vi "Teleop.vi"(10 "Match Info":T2={"Autonomous Elapsed Seconds"=0.0, "TeleOp Elapsed Seconds"=0.0, "Disabled Elapsed Seconds"=0.0, "Visited Autonomous"=FALSE, "Visited TeleOp"=FALSE, "Visited Disabled"=FALSE, "Autonomous Settings"={"Autonomous Style"=enum."Independent", "VI Refnum"=refnum}}, 11 "Call Context":T3) -> ()   [LabVIEW 2017]
doc: "This VI is called for each TeleOp packet received from the DS where the robot is not disabled. It is often used to read from the joysticks and update I/O or to update setpoints for timed control loops. It should complete and return within 20 milliseconds or it may miss DS packets."
uses:
  <vilib>/Rock Robotics/WPI/DriverStation/WPI_DriverStationDerivedRobotMode.ctl
  <vilib>/Rock Robotics/WPI/DriverStation/WPI_DriverStationMatch Info.ctl
  <vilib>/Rock Robotics/WPI/Solenoid/WPI_SolenoidValue.ctl
  <vilib>/Rock Robotics/WPI/Utilities/WPI_GetSetVariantRefNum.vi
  <vilib>/Rock Robotics/WPI/RobotDrive/WPI_RobotDriveMecanumDrive_Cartesian.vi
  <vilib>/Rock Robotics/Network Tables/NT Write Numeric Array.vi
  <vilib>/Rock Robotics/WPI/Solenoid/WPI_SolenoidSetEnum.vi
  Robot Global Data.vi
  <vilib>/Rock Robotics/Network Tables/NT Write Number.vi
panel:
  out "Stopped":bool
  out "Rate":dbl
  out "Direction":bool
  out "Distance":dbl
  out "Accelerations":T1
  out "Switch Pressed":bool
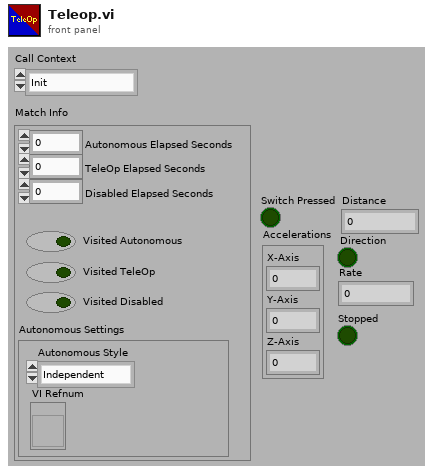
[diagram p1: front panel]
types:
  T1 = cluster{"X-Axis":dbl, "Y-Axis":dbl, "Z-Axis":dbl}
  T2 = typedef "WPI_DriverStationMatch Info.ctl" = cluster{"Autonomous Elapsed Seconds":dbl, "TeleOp Elapsed Seconds":dbl, "Disabled Elapsed Seconds":dbl, "Visited Autonomous":bool, "Visited TeleOp":bool, "Visited Disabled":bool, "Autonomous Settings":cluster{"Autonomous Style":enum16{"Iterative", "Independent"}, "VI Refnum":refnum<vi>}}
  T3 = typedef "WPI_DriverStationDerivedRobotMode.ctl" = enum16{"Init", "Execute", "Stop"}
  T4 = typedef "WPI_SolenoidValue.ctl" = enum16{"Off", "On", "Forward", "Reverse"}
  T5 = typedef "WPI_JoystickDevRef.ctl" = cluster{"Device":T6}
  T6 = typedef "WPI_JoystickDeviceEnum.ctl" = enum16{"USB 0", "USB 1", "USB 2", "USB 3", "USB 4", "USB 5"}
  T7 = typedef "WPI_MotorControlDeviceRef.ctl" = cluster{"DeviceStatus":errorcluster, "Type":T8, "PWM":cluster{"PWM Channel":T9, "DeadBand":T10}, "CAN":cluster{"Device Number":u8, "SetOutput VI Ref":variant, "GetOutput VI Ref":variant, "Enable VI Ref":variant, "Disable VI Ref":variant, "Data":variant}, "Invert":bool, "DIO PWM":cluster{"PWM \"Enable\" Channel":T9, "DIOChannel":T11, "PWM Rate":dbl}}
  T8 = typedef "WPI_MotorControlType.ctl" = enum16{"PWM", "CAN", "DIO PWM"}
  T9 = typedef "FPGA_DIOPWMChannel.ctl" = enum8{"PWM 0", "PWM 1", "PWM 2", "PWM 3", "PWM 4", "PWM 5", "PWM 6", "PWM 7", "PWM 8", "PWM 9", "PWM MXP 0", "PWM MXP 1", "PWM MXP 2", "PWM MXP 3", "PWM MXP 4", "PWM MXP 5", "PWM MXP 6", "PWM MXP 7", "PWM MXP 8", "PWM MXP 9", "Invalid"}
  T10 = typedef "WPI_PWMDeadband.ctl" = cluster{"Name":string, "maxPositivePwm":i32, "minPositivePwm":i32, "centerPwm":i32, "maxNegativePwm":i32, "minNegativePwm":i32, "angularRange":u16}
  T11 = typedef "FPGA_DIOChannel.ctl" = enum8{"DIO 0", "DIO 1", "DIO 2", "DIO 3", "DIO 4", "DIO 5", "DIO 6", "DIO 7", "DIO 8", "DIO 9", "DIO MXP 0", "DIO MXP 1", "DIO MXP 2", "DIO MXP 3", "DIO MXP 4", "DIO MXP 5", "DIO MXP 6", "DIO MXP 7", "DIO MXP 8", "DIO MXP 9", "DIO MXP 10", "DIO MXP 11", "DIO MXP 12", "DIO MXP 13", "DIO MXP 14", "DIO MXP 15", "SPI Port CS1", "SPI Port CS2", "SPI Port CS3", "SPI Port MISO", "SPI Port MOSI", "Invalid"}
  T12 = typedef "WPI_SolenoidDevRef.ctl" = cluster{"DevStatus":errorcluster, "Pneumatics Control Module":u8, "Forward Solenoid Channel":T13, "Reverse Solenoid Channel":T13}
  T13 = typedef "WPI_SolenoidChannel.ctl" = enum8{"Solenoid 0", "Solenoid 1", "Solenoid 2", "Solenoid 3", "Solenoid 4", "Solenoid 5", "Solenoid 6", "Solenoid 7", "Invalid"}
  T14 = typedef "WPI_RobotDriveDevRef.ctl" = cluster{"DevStatus":errorcluster, "Motors[]":T7[], "Square Inputs":bool, "Max Output":dbl}
  T15 = typedef "WPI_SwitchDevRef.ctl" = cluster{"DevStatus":errorcluster, "DIO Channel":T11, "CntIndex":T16, "Normally Closed":bool}
  T16 = typedef "FPGA_CounterCtrSystemIndex.ctl" = enum8{"Ctr 0", "Ctr 1", "Ctr 2", "Ctr 3", "Ctr 4", "Ctr 5", "Ctr 6", "Ctr 7", "Invalid"}
  T17 = typedef "WPI_AccelerometerDevRef.ctl" = cluster{"DevStatus":errorcluster, "Scaling":T18, "Analog Channels":T19, "I2C Bus":T21, "SPI Bus":T22, "Accel Range":T23, "ADXL Axes":T24, "Handle":i32, "Device Address":u8, "Accel Type":enum16{"Analog", "ADXL345 I2C", "ADXL345 SPI", "Internal", "ADXL362 SPI"}}
  T18 = typedef "WPI_AccelerometerScaling.ctl" = cluster{"Gain (VoltsPerG)":dbl, "Center Voltage":dbl}
  T19 = typedef "WPI_AccelerometerAnalogChannels.ctl" = cluster{"X-Axis":T20, "Y-Axis":T20, "Z-Axis":T20}
  T20 = typedef "FPGA_AIChannel.ctl" = enum8{"AI 0", "AI 1", "AI 2", "AI 3", "AI MXP 0", "AI MXP 1", "AI MXP 2", "AI MXP 3", "Invalid"}
  T21 = typedef "i2c_bus.ctl" = enum16{"I2C On-Board", "I2C MXP", "Invalid"}
  T22 = typedef "spi_bus.ctl" = enum16{"SPI On-Board, CS0", "SPI On-Board, CS1", "SPI On-Board, CS2", "SPI On-Board, CS3", "SPI MXP", "Invalid"}
  T23 = typedef "ADXL345 Range.ctl" = u8
  T24 = typedef "WPI_AccelerometerADXL345 Axes.ctl" = cluster{"X-Axis":bool, "Y-Axis":bool, "Z-Axis":bool}
  T25 = typedef "WPI_EncoderDevRef.ctl" = cluster{"DevStatus":errorcluster, "EncoderIndex":T26, "CounterIndex":T16, "DistancePerCount":dbl, "Decoding Type":T27}
  T26 = typedef "FPGA_EncoderIdx.ctl" = enum8{"Enc 0", "Enc 1", "Enc 2", "Enc 3", "Enc 4", "Enc 5", "Enc 6", "Enc 7", "Invalid"}
  T27 = typedef "WPI_EncoderType.ctl" = enum16{"1x", "2x", "4x"}
  T28 = typedef "WPI_GyroDevRef.ctl" = cluster{"DevStatus":errorcluster, "Analog Channel":T20, "Gain (VoltsPerDegree/Second)":dbl, "Gyro Type":enum16{"Analog", "XRS450"}, "Handle":i32, "SPI Bus":T22, "Device Found":bool, "Sample Rate":dbl, "Calibrate On Open":bool, "Offset":dbl}
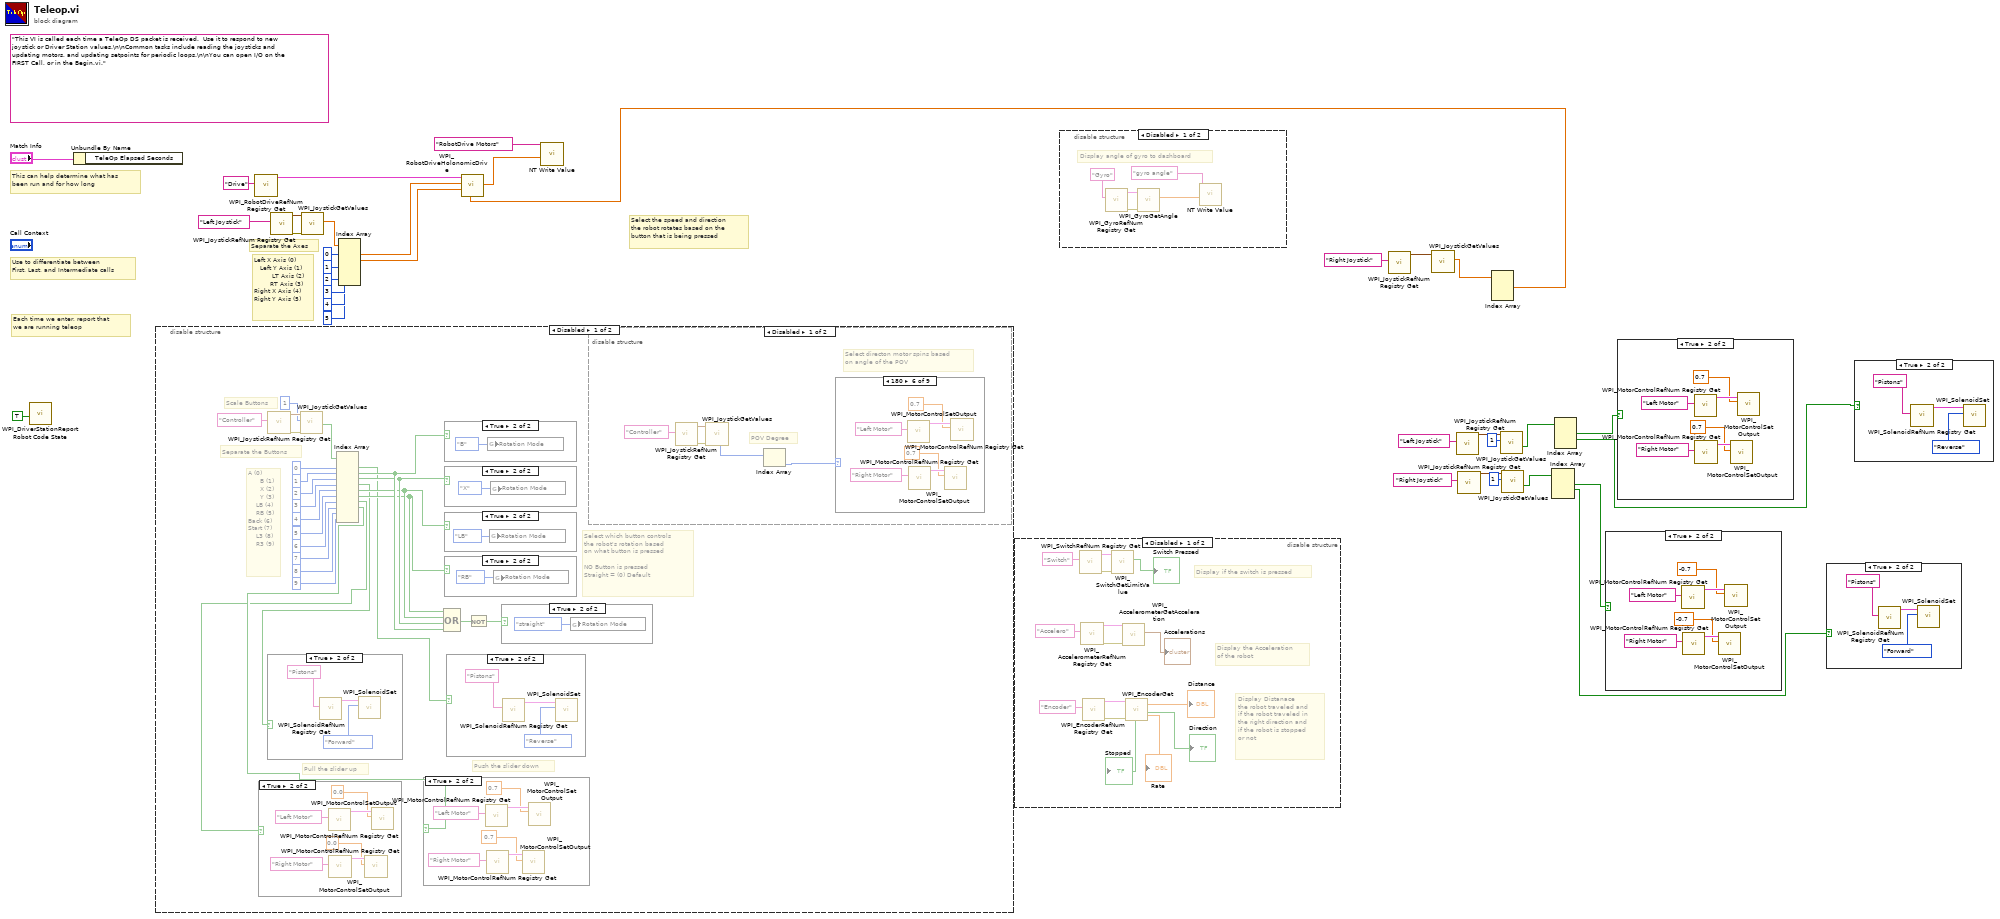
[diagram p0: block diagram]
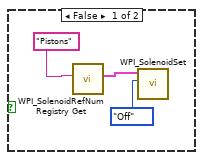
[diagram p2: hidden frame]
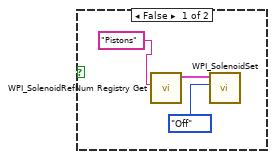
[diagram p3: hidden frame]
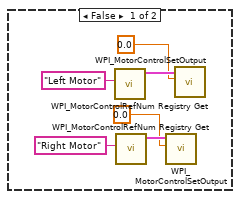
[diagram p4: hidden frame]
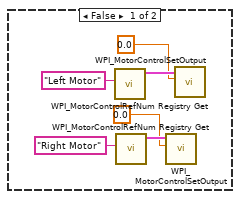
[diagram p5: hidden frame]
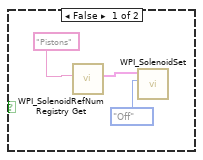
[diagram p8: hidden frame]
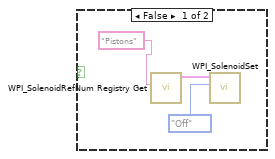
[diagram p9: hidden frame]
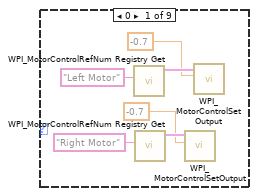
[diagram p15: hidden frame]
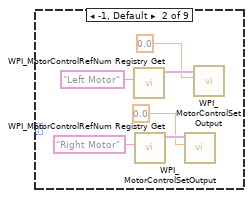
[diagram p16: hidden frame]
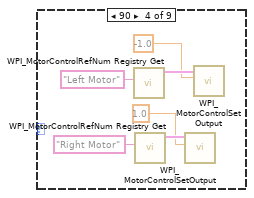
[diagram p18: hidden frame]
diagram:
  (unwired) "This VI is called each time a TeleOp DS packet is received.  Use it to respond to new joystick or Driver Station values.\n\nCommon tasks include reading the joysticks and updating motors, and updating setpoints for periodic loops.\n\nYou can open I/O on the FIRST Call, or in the Begin.vi."
  # "Select the speed and direction\nthe robot rotates based on the \nbutton that is being pressed"
  # "Left X Axis (0)\n   Left Y Axis (1)\n         LT Axis (2)\n        RT Axis (3)\nRight X Axis (4)\nRight Y Axis (5)"
  # "Separate the Axes"
  # "Each time we enter, report that\nwe are running teleop"
  # "Use to differentiate between\nFirst, Last, and Intermediate calls"
  # "This can help determine what has\nbeen run and for how long"
  n1 = call <vilib>:"WPI_DriverStationReport Robot Code State.vi"("TeleOp"=TRUE ("Autonomous")) -> ()  [unwired: 10 in, 1 out]
  n2 = Unbundle By Name("Match Info") -> ()  [unwired: 1 out]
  n3 = disable-structure shown="Disabled" {
    frame Disabled {
      # "Select which button controls\nthe robot's rotation based\non what button is pressed\n\nNO Button is pressed\nStraight = (0) Default"
      # "Pull the slider up"
      # "Push the slider down"
      # "A (0)\n      B (1)\n      X (2)\n      Y (3)\n    LB (4)\n    RB (5)\nBack (6)\nStart (7)\n    L3 (8)\n    R3 (9)"
      # "Separate the Buttons"
      # "Scale Buttons"
      n4 = call <vilib>:"WPI_JoystickRefNum Registry Get.vi"("refnum name"="Controller") -> ("error out"=w59:errorcluster, "JoystickDevRef"=w58:T5)  [unwired: 9 in]
      n5 = call <vilib>:"WPI_JoystickGetValues.vi"("error in (no error)"=w59, "Scaler"=i8 1, "JoystickDevRef"=w58) -> ("Buttons"=w37:bool[])  [unwired: 4 in, 4 out]
      n6 = Index Array(array=w37, index #1=0 ("index"), index #2=1 ("index"), index #3=2 ("index"), index #4=3 ("index"), index #5=4 ("index"), index #6=5 ("index"), index #7=6 ("index"), index #8=7 ("index"), index #9=8 ("index"), index #10=9 ("index")) -> (element #1=w39:bool, element #2=w43:bool, element #3=w42:bool, element #4=w38:bool, element #5=w41:bool, element #6=w40:bool, element #7=w35:bool, element #8=w36:bool)  [unwired: 2 out]
      n7 = case shown="True" w35 {
        frame False {
        }
        frame True {
          n8 = call <vilib>:"WPI_MotorControlRefNum Registry Get.vi"("refnum name"="Left Motor") -> ("MotorControlDevRef"=w70:T7)  [unwired: 9 in, 1 out]
          n9 = call <vilib>:"WPI_MotorControlRefNum Registry Get.vi"("refnum name"="Right Motor") -> ("MotorControlDevRef"=w71:T7)  [unwired: 9 in, 1 out]
          n10 = call <vilib>:"WPI_MotorControlSetOutput.vi"("Output"=0.0, "MotorControlDevRef"=w71) -> ()  [unwired: 7 in, 3 out]
          n11 = call <vilib>:"WPI_MotorControlSetOutput.vi"("Output"=0.0, "MotorControlDevRef"=w70) -> ()  [unwired: 7 in, 3 out]
        }
      }
      n12 = case shown="True" w38 {
        frame False {
          n13 = call <vilib>:"WPI_SolenoidRefNum Registry Get.vi"("refnum name"="Pistons") -> ("SolenoidDevRef"=w74:T12)  [unwired: 9 in, 1 out]
          n14 = call-poly <vilib>:"WPI_SolenoidSet.vi"("Value"=WPI_SolenoidValue."Off", "SolenoidDevRef"=w74) -> ()  [unwired: 8 in, 2 out]
        }
        frame True {
          n15 = call <vilib>:"WPI_SolenoidRefNum Registry Get.vi"("refnum name"="Pistons") -> ("SolenoidDevRef"=w76:T12)  [unwired: 9 in, 1 out]
          n16 = call-poly <vilib>:"WPI_SolenoidSet.vi"("Value"=WPI_SolenoidValue."Forward", "SolenoidDevRef"=w76) -> ()  [unwired: 8 in, 2 out]
        }
      }
      n17 = case shown="True" w36 {
        frame False {
        }
        frame True {
          n18 = call <vilib>:"WPI_MotorControlRefNum Registry Get.vi"("refnum name"="Left Motor") -> ("MotorControlDevRef"=w64:T7)  [unwired: 9 in, 1 out]
          n19 = call <vilib>:"WPI_MotorControlRefNum Registry Get.vi"("refnum name"="Right Motor") -> ("MotorControlDevRef"=w62:T7)  [unwired: 9 in, 1 out]
          n20 = call <vilib>:"WPI_MotorControlSetOutput.vi"("Output"=0.7, "MotorControlDevRef"=w62) -> ()  [unwired: 7 in, 3 out]
          n21 = call <vilib>:"WPI_MotorControlSetOutput.vi"("Output"=0.7, "MotorControlDevRef"=w64) -> ()  [unwired: 7 in, 3 out]
        }
      }
      n22 = Compound Arithmetic op=OR(w40, w41, w42, w43) -> (w55:bool)
      n23 = case shown="True" w43 {
        frame False {
        }
        frame True {
          n24 = global write "Robot Global Data.vi" "Rotation Mode"(enum16{"straight", "X", "LB", "B", "RB"}."B" ("Rotation Mode")) -> ()
        }
      }
      n25 = case shown="True" w42 {
        frame False {
        }
        frame True {
          n26 = global write "Robot Global Data.vi" "Rotation Mode"(enum16{"straight", "X", "LB", "B", "RB"}."X" ("Rotation Mode")) -> ()
        }
      }
      n27 = case shown="True" w41 {
        frame False {
        }
        frame True {
          n28 = global write "Robot Global Data.vi" "Rotation Mode"(enum16{"straight", "X", "LB", "B", "RB"}."LB" ("Rotation Mode")) -> ()
        }
      }
      n29 = case shown="True" w40 {
        frame False {
        }
        frame True {
          n30 = global write "Robot Global Data.vi" "Rotation Mode"(enum16{"straight", "X", "LB", "B", "RB"}."RB" ("Rotation Mode")) -> ()
        }
      }
      n31 = case shown="True" w39 {
        frame False {
          n32 = call <vilib>:"WPI_SolenoidRefNum Registry Get.vi"("refnum name"="Pistons") -> ("SolenoidDevRef"=w80:T12)  [unwired: 9 in, 1 out]
          n33 = call-poly <vilib>:"WPI_SolenoidSet.vi"("Value"=WPI_SolenoidValue."Off", "SolenoidDevRef"=w80) -> ()  [unwired: 8 in, 2 out]
        }
        frame True {
          n34 = call <vilib>:"WPI_SolenoidRefNum Registry Get.vi"("refnum name"="Pistons") -> ("SolenoidDevRef"=w82:T12)  [unwired: 9 in, 1 out]
          n35 = call-poly <vilib>:"WPI_SolenoidSet.vi"("Value"=WPI_SolenoidValue."Reverse", "SolenoidDevRef"=w82) -> ()  [unwired: 8 in, 2 out]
        }
      }
      n36 = Not(x=w55) -> (.not. x?=w54:bool)
      n37 = case shown="True" w54 {
        frame False {
        }
        frame True {
          n38 = global write "Robot Global Data.vi" "Rotation Mode"(enum16{"straight", "X", "LB", "B", "RB"}."straight" ("Rotation Mode")) -> ()
        }
      }
      n39 = disable-structure shown="Disabled" {
        frame Disabled {
          # "Select directon motor spins based\non angle of the POV"
          # "POV Degree"
          n40 = call <vilib>:"WPI_JoystickRefNum Registry Get.vi"("refnum name"="Controller") -> ("error out"=w93:errorcluster, "JoystickDevRef"=w92:T5)  [unwired: 9 in]
          n41 = call <vilib>:"WPI_JoystickGetValues.vi"("error in (no error)"=w93, "JoystickDevRef"=w92) -> ("POVs"=w90:i16[])  [unwired: 5 in, 4 out]
          n42 = Index Array(array=w90) -> (element=w89:i16)  [unwired: 1 in]
          n43 = case shown="180" w89 {
            frame 0 {
              n44 = call <vilib>:"WPI_MotorControlRefNum Registry Get.vi"("refnum name"="Left Motor") -> ("MotorControlDevRef"=w98:T7)  [unwired: 9 in, 1 out]
              n45 = call <vilib>:"WPI_MotorControlRefNum Registry Get.vi"("refnum name"="Right Motor") -> ("MotorControlDevRef"=w96:T7)  [unwired: 9 in, 1 out]
              n46 = call <vilib>:"WPI_MotorControlSetOutput.vi"("Output"=-0.7, "MotorControlDevRef"=w96) -> ()  [unwired: 7 in, 3 out]
              n47 = call <vilib>:"WPI_MotorControlSetOutput.vi"("Output"=-0.7, "MotorControlDevRef"=w98) -> ()  [unwired: 7 in, 3 out]
            }
            frame -1, Default {
              n48 = call <vilib>:"WPI_MotorControlRefNum Registry Get.vi"("refnum name"="Left Motor") -> ("MotorControlDevRef"=w104:T7)  [unwired: 9 in, 1 out]
              n49 = call <vilib>:"WPI_MotorControlRefNum Registry Get.vi"("refnum name"="Right Motor") -> ("MotorControlDevRef"=w102:T7)  [unwired: 9 in, 1 out]
              n50 = call <vilib>:"WPI_MotorControlSetOutput.vi"("Output"=0.0, "MotorControlDevRef"=w102) -> ()  [unwired: 7 in, 3 out]
              n51 = call <vilib>:"WPI_MotorControlSetOutput.vi"("Output"=0.0, "MotorControlDevRef"=w104) -> ()  [unwired: 7 in, 3 out]
            }
            frame 45 {
            }
            frame 90 {
              n52 = call <vilib>:"WPI_MotorControlRefNum Registry Get.vi"("refnum name"="Left Motor") -> ("MotorControlDevRef"=w110:T7)  [unwired: 9 in, 1 out]
              n53 = call <vilib>:"WPI_MotorControlRefNum Registry Get.vi"("refnum name"="Right Motor") -> ("MotorControlDevRef"=w108:T7)  [unwired: 9 in, 1 out]
              n54 = call <vilib>:"WPI_MotorControlSetOutput.vi"("Output"=1.0, "MotorControlDevRef"=w108) -> ()  [unwired: 7 in, 3 out]
              n55 = call <vilib>:"WPI_MotorControlSetOutput.vi"("Output"=-1.0, "MotorControlDevRef"=w110) -> ()  [unwired: 7 in, 3 out]
            }
            frame 135 {
            }
            frame 180 {
              n56 = call <vilib>:"WPI_MotorControlRefNum Registry Get.vi"("refnum name"="Left Motor") -> ("MotorControlDevRef"=w116:T7)  [unwired: 9 in, 1 out]
              n57 = call <vilib>:"WPI_MotorControlRefNum Registry Get.vi"("refnum name"="Right Motor") -> ("MotorControlDevRef"=w114:T7)  [unwired: 9 in, 1 out]
              n58 = call <vilib>:"WPI_MotorControlSetOutput.vi"("Output"=0.7, "MotorControlDevRef"=w114) -> ()  [unwired: 7 in, 3 out]
              n59 = call <vilib>:"WPI_MotorControlSetOutput.vi"("Output"=0.7, "MotorControlDevRef"=w116) -> ()  [unwired: 7 in, 3 out]
            }
            frame 225 {
            }
            frame 270 {
              n60 = call <vilib>:"WPI_MotorControlRefNum Registry Get.vi"("refnum name"="Left Motor") -> ("MotorControlDevRef"=w122:T7)  [unwired: 9 in, 1 out]
              n61 = call <vilib>:"WPI_MotorControlRefNum Registry Get.vi"("refnum name"="Right Motor") -> ("MotorControlDevRef"=w120:T7)  [unwired: 9 in, 1 out]
              n62 = call <vilib>:"WPI_MotorControlSetOutput.vi"("Output"=-1.0, "MotorControlDevRef"=w120) -> ()  [unwired: 7 in, 3 out]
              n63 = call <vilib>:"WPI_MotorControlSetOutput.vi"("Output"=1.0, "MotorControlDevRef"=w122) -> ()  [unwired: 7 in, 3 out]
            }
            frame 315 {
            }
          }
        }
        frame Enabled {
        }
      }
    }
    frame Enabled {
    }
  }
  n64 = call <vilib>:"WPI_RobotDriveRefNum Registry Get.vi"("refnum name"="Drive") -> ("RobotDriveDevRef"=w27:T14)  [unwired: 9 in, 1 out]
  n65 = call <vilib>:"WPI_JoystickRefNum Registry Get.vi"("refnum name"="Left Joystick") -> ("error out"=w31:errorcluster, "JoystickDevRef"=w30:T5)  [unwired: 9 in]
  n66 = call <vilib>:"WPI_JoystickGetValues.vi"("error in (no error)"=w31, "JoystickDevRef"=w30) -> ("Axes"=w29:dbl[])  [unwired: 5 in, 4 out]
  n67 = Index Array(array=w29, index #1=0 ("index"), index #2=1 ("index"), index #3=2 ("index"), index #4=3 ("index"), index #5=4 ("index"), index #6=5 ("index")) -> (element #1=w26:dbl, element #2=w25:dbl)  [unwired: 4 out]
  n68 = disable-structure shown="Disabled" {
    frame Disabled {
      # "Display Distanace\nthe robot traveled and\nif the robot traveled in \nthe right direction and\nif the robot is stopped \nor not"
      # "Display the Acceleration\nof the robot"
      # "Display if the switch is pressed"
      n69 = call <vilib>:"WPI_SwitchRefNum Registry Get.vi"("refnum name"="Switch") -> ("error out"=w137:errorcluster, "SwitchDevRef"=w136:T15)  [unwired: 9 in]
      n70 = call <vilib>:"WPI_AccelerometerRefNum Registry Get.vi"("refnum name"="Accelero") -> ("error out"=w134:errorcluster, "AccelerometerDevRef"=w133:T17)  [unwired: 9 in]
      n71 = call <vilib>:"WPI_EncoderRefNum Registry Get.vi"("refnum name"="Encoder") -> ("error out"=w129:errorcluster, "EncoderDevRef"=w128:T25)  [unwired: 9 in]
      n72 = call <vilib>:"WPI_SwitchGetLimitValue.vi"("error in (no error)"=w137, "SwitchDevRef"=w136) -> ("Switch Pressed"=→"Switch Pressed":bool)  [unwired: 7 in, 2 out]
      n73 = call <vilib>:"WPI_AccelerometerGetAcceleration.vi"("error in"=w134, "AccelerometerDevRef"=w133) -> ("Accelerations"=→"Accelerations":T1)  [unwired: 7 in, 2 out]
      n74 = call <vilib>:"WPI_EncoderGet.vi"("error in (no error)"=w129, "EncoderDevRef"=w128) -> ("Direction"=→"Direction":bool, "Distance"=→"Distance":dbl, "Rate"=→"Rate":dbl, "Stopped"=→"Stopped":bool)  [unwired: 4 in, 2 out]
    }
    frame Enabled {
    }
  }
  n75 = disable-structure shown="Disabled" {
    frame Disabled {
      # "Display angle of gyro to dashboard"
      n76 = call <vilib>:"WPI_GyroRefNum Registry Get.vi"("refnum name"="Gyro") -> ("error out"=w142:errorcluster, "GyroDevRef"=w141:T28)  [unwired: 9 in]
      n77 = call <vilib>:"WPI_GyroGetAngle.vi"("error in"=w142, "GyroDevRef"=w141) -> ("Angle"=w139:dbl)  [unwired: 5 in, 4 out]
      n78 = call-poly <vilib>:"NT Write Value.vi"("Numeric"=w139, "Name"="gyro angle") -> ()  [unwired: 9 in, 1 out]
    }
    frame Enabled {
    }
  }
  n79 = call <vilib>:"WPI_JoystickRefNum Registry Get.vi"("refnum name"="Right Joystick") -> ("JoystickDevRef"=w15:T5)  [unwired: 9 in, 1 out]
  n80 = call <vilib>:"WPI_JoystickGetValues.vi"("JoystickDevRef"=w15) -> ("Axes"=w14:dbl[])  [unwired: 6 in, 4 out]
  n81 = call <vilib>:"WPI_JoystickRefNum Registry Get.vi"("refnum name"="Left Joystick") -> ("JoystickDevRef"=w9:T5)  [unwired: 9 in, 1 out]
  n82 = call <vilib>:"WPI_JoystickRefNum Registry Get.vi"("refnum name"="Right Joystick") -> ("JoystickDevRef"=w11:T5)  [unwired: 9 in, 1 out]
  n83 = Index Array(array=w14) -> (element #1=w13:dbl)  [unwired: 3 in, 2 out]
  n84 = call-poly <vilib>:"WPI_RobotDriveHolonomicDrive.vi"("Rotation"=w13, "Y"=w25, "X"=w26, "RobotDriveDevRef"=w27) -> ("Motor Values"=w24:dbl[])  [unwired: 5 in, 2 out]
  n85 = call-poly <vilib>:"NT Write Value.vi"("Numeric Array"=w24, "Name"="RobotDrive Motors") -> ()  [unwired: 9 in, 1 out]
  n86 = call <vilib>:"WPI_JoystickGetValues.vi"("Scaler"=i8 1, "JoystickDevRef"=w9) -> ("Buttons"=w6:bool[])  [unwired: 5 in, 4 out]
  n87 = call <vilib>:"WPI_JoystickGetValues.vi"("Scaler"=i8 1, "JoystickDevRef"=w11) -> ("Buttons"=w5:bool[])  [unwired: 5 in, 4 out]
  n88 = Index Array(array=w5) -> (element #1=w4:bool, element #2=w1:bool)  [unwired: 3 in, 1 out]
  n89 = Index Array(array=w6) -> (element #1=w3:bool, element #2=w2:bool)  [unwired: 3 in, 1 out]
  n90 = case shown="True" w4 {
    frame False {
      n91 = call <vilib>:"WPI_MotorControlRefNum Registry Get.vi"("refnum name"="Left Motor") -> ("MotorControlDevRef"=w148:T7)  [unwired: 9 in, 1 out]
      n92 = call <vilib>:"WPI_MotorControlRefNum Registry Get.vi"("refnum name"="Right Motor") -> ("MotorControlDevRef"=w149:T7)  [unwired: 9 in, 1 out]
      n93 = call <vilib>:"WPI_MotorControlSetOutput.vi"("Output"=0.0, "MotorControlDevRef"=w149) -> ()  [unwired: 7 in, 3 out]
      n94 = call <vilib>:"WPI_MotorControlSetOutput.vi"("Output"=0.0, "MotorControlDevRef"=w148) -> ()  [unwired: 7 in, 3 out]
    }
    frame True {
      n95 = call <vilib>:"WPI_MotorControlRefNum Registry Get.vi"("refnum name"="Left Motor") -> ("MotorControlDevRef"=w154:T7)  [unwired: 9 in, 1 out]
      n96 = call <vilib>:"WPI_MotorControlRefNum Registry Get.vi"("refnum name"="Right Motor") -> ("MotorControlDevRef"=w152:T7)  [unwired: 9 in, 1 out]
      n97 = call <vilib>:"WPI_MotorControlSetOutput.vi"("Output"=-0.7, "MotorControlDevRef"=w152) -> ()  [unwired: 7 in, 3 out]
      n98 = call <vilib>:"WPI_MotorControlSetOutput.vi"("Output"=-0.7, "MotorControlDevRef"=w154) -> ()  [unwired: 7 in, 3 out]
    }
  }
  n99 = case shown="True" w3 {
    frame False {
      n100 = call <vilib>:"WPI_MotorControlRefNum Registry Get.vi"("refnum name"="Left Motor") -> ("MotorControlDevRef"=w160:T7)  [unwired: 9 in, 1 out]
      n101 = call <vilib>:"WPI_MotorControlRefNum Registry Get.vi"("refnum name"="Right Motor") -> ("MotorControlDevRef"=w161:T7)  [unwired: 9 in, 1 out]
      n102 = call <vilib>:"WPI_MotorControlSetOutput.vi"("Output"=0.0, "MotorControlDevRef"=w161) -> ()  [unwired: 7 in, 3 out]
      n103 = call <vilib>:"WPI_MotorControlSetOutput.vi"("Output"=0.0, "MotorControlDevRef"=w160) -> ()  [unwired: 7 in, 3 out]
    }
    frame True {
      n104 = call <vilib>:"WPI_MotorControlRefNum Registry Get.vi"("refnum name"="Left Motor") -> ("MotorControlDevRef"=w166:T7)  [unwired: 9 in, 1 out]
      n105 = call <vilib>:"WPI_MotorControlRefNum Registry Get.vi"("refnum name"="Right Motor") -> ("MotorControlDevRef"=w164:T7)  [unwired: 9 in, 1 out]
      n106 = call <vilib>:"WPI_MotorControlSetOutput.vi"("Output"=0.7, "MotorControlDevRef"=w164) -> ()  [unwired: 7 in, 3 out]
      n107 = call <vilib>:"WPI_MotorControlSetOutput.vi"("Output"=0.7, "MotorControlDevRef"=w166) -> ()  [unwired: 7 in, 3 out]
    }
  }
  n108 = case shown="True" w1 {
    frame False {
      n109 = call <vilib>:"WPI_SolenoidRefNum Registry Get.vi"("refnum name"="Pistons") -> ("SolenoidDevRef"=w170:T12)  [unwired: 9 in, 1 out]
      n110 = call-poly <vilib>:"WPI_SolenoidSet.vi"("Value"=WPI_SolenoidValue."Off", "SolenoidDevRef"=w170) -> ()  [unwired: 8 in, 2 out]
    }
    frame True {
      n111 = call <vilib>:"WPI_SolenoidRefNum Registry Get.vi"("refnum name"="Pistons") -> ("SolenoidDevRef"=w172:T12)  [unwired: 9 in, 1 out]
      n112 = call-poly <vilib>:"WPI_SolenoidSet.vi"("Value"=WPI_SolenoidValue."Forward", "SolenoidDevRef"=w172) -> ()  [unwired: 8 in, 2 out]
    }
  }
  n113 = case shown="True" w2 {
    frame False {
      n114 = call <vilib>:"WPI_SolenoidRefNum Registry Get.vi"("refnum name"="Pistons") -> ("SolenoidDevRef"=w176:T12)  [unwired: 9 in, 1 out]
      n115 = call-poly <vilib>:"WPI_SolenoidSet.vi"("Value"=WPI_SolenoidValue."Off", "SolenoidDevRef"=w176) -> ()  [unwired: 8 in, 2 out]
    }
    frame True {
      n116 = call <vilib>:"WPI_SolenoidRefNum Registry Get.vi"("refnum name"="Pistons") -> ("SolenoidDevRef"=w178:T12)  [unwired: 9 in, 1 out]
      n117 = call-poly <vilib>:"WPI_SolenoidSet.vi"("Value"=WPI_SolenoidValue."Reverse", "SolenoidDevRef"=w178) -> ()  [unwired: 8 in, 2 out]
    }
  }
